vi "CTRE_Phoenix_Pigeon2_GetStatus.vi"   [LabVIEW 2020]
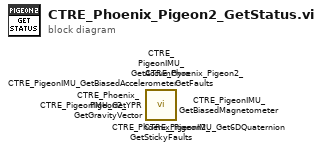
[diagram p0: block diagram]
diagram:
  n1 = call <vilib>:"CTRE_Phoenix_Pigeon2_GetStickyFaults.vi"() -> ()  [unwired: 9 in, 3 out]
  n2 = call <vilib>:"CTRE_Phoenix_Pigeon2_GetFaults.vi"() -> ()  [unwired: 9 in, 3 out]
  n3 = call <vilib>:"CTRE_PigeonIMU_GetYPR.vi"() -> ()  [unwired: 9 in, 3 out]
  n4 = call <vilib>:"CTRE_PigeonIMU_GetBiasedMagnetometer.vi"() -> ()  [unwired: 9 in, 3 out]
  n5 = call <vilib>:"CTRE_PigeonIMU_GetBiasedAccelerometer.vi"() -> ()  [unwired: 9 in, 3 out]
  n6 = call <vilib>:"CTRE_PigeonIMU_GetAccumGyro.vi"() -> ()  [unwired: 9 in, 3 out]
  n7 = call <vilib>:"CTRE_PigeonIMU_Get6DQuaternion.vi"() -> ()  [unwired: 9 in, 3 out]
  n8 = call <vilib>:"CTRE_Phoenix_Pigeon2_GetGravityVector.vi"() -> ()  [unwired: 9 in, 3 out]
